vi "Init.vi"(8 "error in":errorcluster, 11 "Scope VISA CFG in":refnum<class "Scope VISA CFG.lvclass">) -> (0 "error out":errorcluster, 3 "Scope VISA CFG out":refnum<class "Scope VISA CFG.lvclass">)   [LabVIEW 2023, in "Scope VISA.lvlib" / "Scope VISA CFG.lvclass"]
uses:
  Scope VISA CFG.lvclass
  Configuration Base/Configuration Base.lvclass/Configuration Base.ctl
  Scope VISA CFG.lvclass/Scope VISA CFG.ctl
  2b7bcb15-04f4-4e40-91e9-05d441e86d6e.vi
  <vilib>/JDP Science/JSONtext/Find Item.vi
  <vilib>/JDP Science/JSONtext/Next JSON Value.vi
  <vilib>/JDP Science/JSONtext/String Subset.vi
  <vilib>/JDP Science/JSONtext/Parsing/Advance past next JSON Value (inlined COPY).vi
  <vilib>/JDP Science/JSONtext/Parsing/Advance past whitespace.vi
  <vilib>/JDP Science/JSONtext/Parsing/Advance past String.vi
  <vilib>/JDP Science/JSONtext/Parsing/Advance past Number.vi
  <vilib>/JDP Science/JSONtext/Parsing/Advance past Line Ending.vi
  <vilib>/JDP Science/JSONtext/Parsing/Parse Full Path or Item Name.vi
  <vilib>/JDP Science/JSONtext/Parsing/Advance past Array.vi
  <vilib>/JDP Science/JSONtext/Parsing/Advance past Object.vi
  <vilib>/JDP Science/JSONtext/support/Error Cluster From Code.vi
  <vilib>/JDP Science/JSONtext/Offset/Find Item Locations by Path.vi
  <vilib>/JDP Science/JSONtext/JSON text to Variant.vi
  <vilib>/Utility/error.llb/Error Cluster From Error Code.vi
  <vilib>/JDP Science/JSONtext/LVClass Serializer/JSONtext LVClass Serializer.lvclass
  <vilib>/ErrorRing/Error Ring.xnode
  Configuration Base/Configuration Base.lvclass
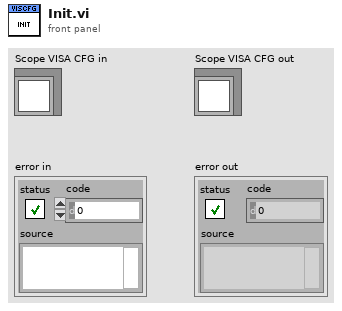
[diagram p1: front panel]
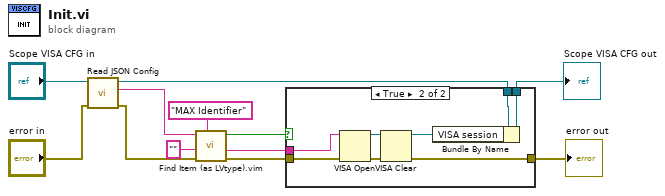
[diagram p0: block diagram]
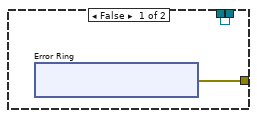
[diagram p2: hidden frame]
diagram:
  n1 = call "Read JSON Config.vi"("error in (no error)"="error in", "object in"="Scope VISA CFG in") -> ("error out"=w9:errorcluster, "<JSON>Config"=w7:string, "object out"=w2:refnum<class "Scope VISA CFG.lvclass">)  [unwired: 7 in]
  n2 = call "Find Item (as LVtype).vim"("$Path or Item Name"="MAX Identifier", "error in (no error)"=w9, "Data Type and Default Value"="", "JSON"=w7) -> ("error out"=w8:errorcluster, "Data"=w4:string, "Found"=w3:bool)  [unwired: 4 in, 1 out]
  n3 = case shown="True" w3 {
    tunnel: [w13 w22] -> w12
    tunnel: w8 -> [_ w26]
    tunnel: w4 -> [_ w25]
    tunnel: w2 -> [w14 w24]
    tunnel: [w14 w23] -> w1
    frame False {
      n4 = xnode "Error Ring"() -> ("error out"=w13:errorcluster)
    }
    frame True {
      n5 = VISA Open(error in (no error)=w26, VISA resource name=w25) -> (VISA resource name=w21:refnum<visa-resource-name>, error out=w27:errorcluster)  [unwired: 3 in]
      n6 = VISA Clear(VISA resource name=w21, error in (no error)=w27) -> (VISA resource name out=w20:refnum<visa-resource-name>, error out=w22:errorcluster)
      n7 = Bundle By Name(cluster=w24, "VISA session"=w20) -> (w23:refnum<class "Scope VISA CFG.lvclass">)
    }
  }
  "error out" <- w12
  "Scope VISA CFG out" <- w1
